vi "Correct.vi"(10 "Input":variant, 11 "Data in":waveform(dbl)[](array[waveform])) -> (1 "Incorrect movement":bool, 2 "Correct movement":bool, 3 "Centered":bool)   [LabVIEW 2010]
uses:
  <vilib>/Analysis/NI_AALBase.lvlib
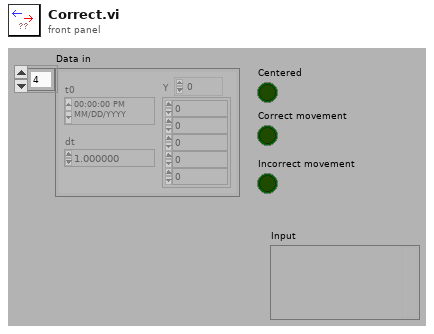
[diagram p1: front panel]
types:
  T1 = cluster{"Trial Type":i32, "Joystick Threshold":dbl, "Fixation Radius":dbl}
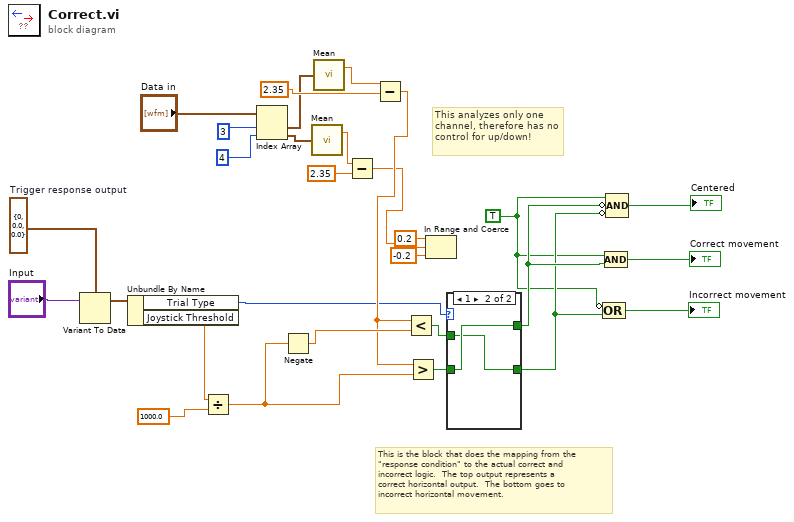
[diagram p0: block diagram]
diagram:
  w1 = T1 {"Trial Type"=0, "Joystick Threshold"=0.0, "Fixation Radius"=0.0}  # Trigger response output
  w16 = TRUE ("value")
  # "This analyzes only one channel, therefore has no control for up/down!"
  # "This is the block that does the mapping from the \n\"response condition\" to the actual correct and \nincorrect logic.  The top output represents a \ncorrect horizontal output.  The bottom goes to\nincorrect horizontal movement."
  n1 = Variant To Data(Variant="Input", type=w1) -> (data=w4:T1)  [unwired: 1 in, 1 out]
  n2 = Unbundle By Name(w4) -> ("Trial Type"=w3:i32, "Joystick Threshold"=w2:dbl)
  n3 = Divide(x=w2, y=1000.0) -> (x/y=w14:dbl)
  n4 = Index Array(array="Data in", index #1=3 ("index"), index #2=4 ("index")) -> (element #1=w11:waveform(dbl), element #2=w9:waveform(dbl))
  n5 = Negate(x=w14) -> (-x=w15:dbl)
  n6 = call <vilib>:"Mean.vi"("X"=w9) -> ("mean"=w8:dbl)  [unwired: 1 out]
  n7 = call <vilib>:"Mean.vi"("X"=w11) -> ("mean"=w10:dbl)  [unwired: 1 out]
  n8 = Subtract(x=w8, y=2.35) -> (x-y=w6:dbl)
  n9 = Subtract(x=w10, y=2.35) -> (x-y=w7:dbl)
  n10 = Less?(x=w7, y=w15) -> (x < y?=w27:bool)
  n11 = Greater?(x=w7, y=w14) -> (0:w26:bool)
  n12 = In Range and Coerce(upper limit=0.2, x=w6, lower limit=-0.2) -> ()  [unwired: 2 out]
  n13 = case shown="1" w3 {
    tunnel: [w31 w33] -> w24
    tunnel: w27 -> [w31 w32]
    tunnel: [w30 w32] -> w22
    tunnel: w26 -> [w30 w33]
    frame 0, Default {
    }
    frame 1 {
    }
  }
  n14 = Compound Arithmetic op=OR(invert w16, w22) -> (→"Incorrect movement":bool)
  n15 = Compound Arithmetic op=AND(w16, w24) -> (→"Correct movement":bool)
  n16 = Compound Arithmetic op=AND(w16, invert w24, invert w22) -> (→"Centered":bool)
